vi "Write queue reference.vi"(8 "error in (no error)":errorcluster, 11 "ALA_Display_Queue ref":refnum<queue>) -> (0 "error out":errorcluster)   [LabVIEW 2020, in "queue_core_loop.lvlib"]
uses:
  queue_core_loop.lvlib
  PTRL/dev_and_debug_tools/QueueMessage typedef.ctl
  library_variable.vi
  PTRL/dev_and_debug_tools/dev_and_debug_tools.lvlib
panel:
  # "Development\ncontrols/indicators useful for development and testing, but which are not outputs of the VI"
  # "Input\nInputs to the VI"
  # "Output\nOutputs of the VI"
  # "Description\n\nBlank VI with error handling case. \n\nSummarize the use of this VI in this space."
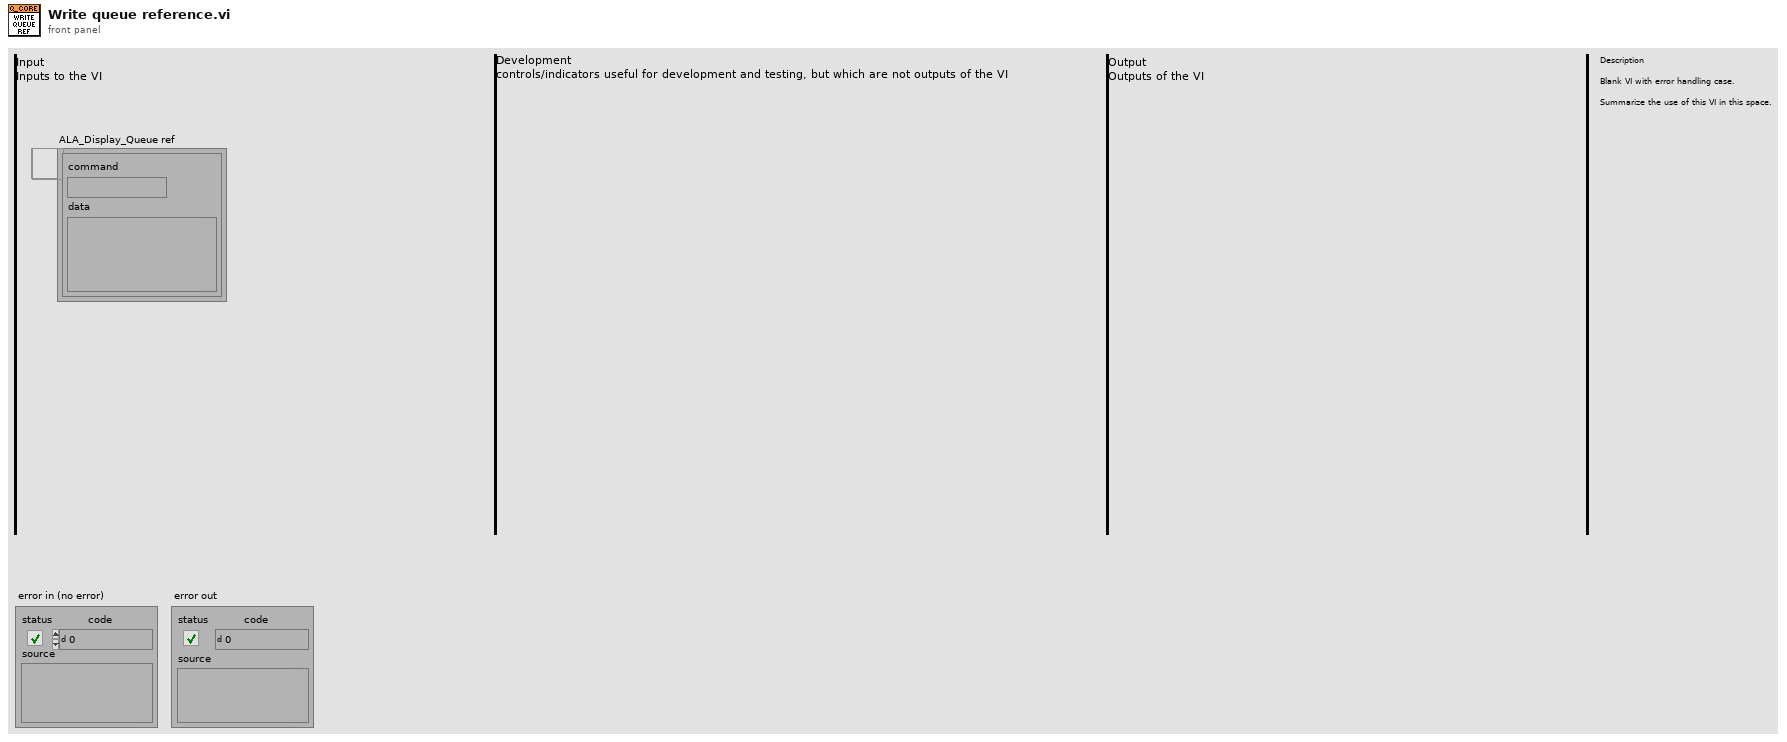
[diagram p1: front panel]
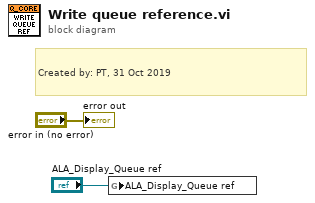
[diagram p0: block diagram]
diagram:
  # "Created by: PT, 31 Oct 2019"
  n1 = global write "library_variable.vi" "ALA_Display_Queue ref"("ALA_Display_Queue ref") -> ()
  "error out" <- "error in (no error)"
